vi "set FPS.vi"(8 "error in (no error)":errorcluster, 11 "Thorcam in":refnum<class "Thorcam.lvclass">) -> (0 "error out":errorcluster, 3 "Thorcam out":refnum<class "Thorcam.lvclass">)   [LabVIEW 2012, in "Thorcam.lvclass"]
uses:
  Thorcam.lvclass
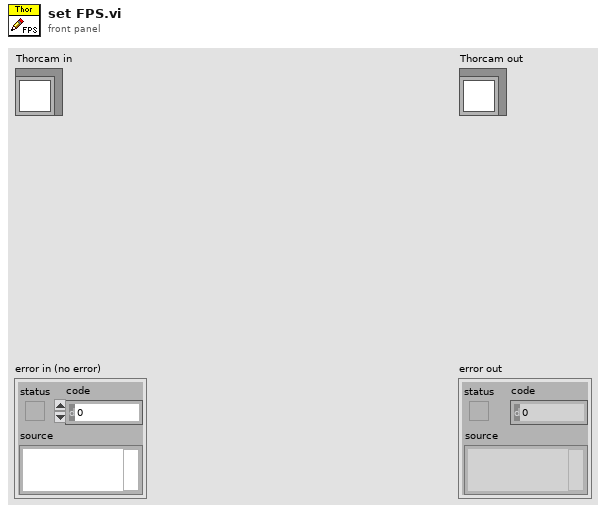
[diagram p1: front panel]
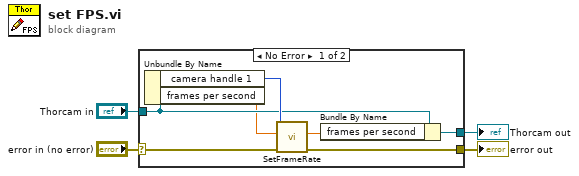
[diagram p0: block diagram]
diagram:
  n1 = case shown="No Error" "error in (no error)" {
    selector: "error in (no error)" -> [w10 w13]
    tunnel: [w9 w13] -> w3
    tunnel: [w7 w12] -> w1
    tunnel: "Thorcam in" -> [w8 w12]
    frame No Error {
      n2 = Unbundle By Name(w8) -> ("camera handle 1"=w11:u32, "frames per second"=w6:dbl)
      n3 = call <instrlib>:"SetFrameRate.vi"("error in"=w10, "FPS"=w6, "Camera Handle In"=w11) -> ("error out"=w9:errorcluster, "new FPS"=w5:dbl)  [unwired: 6 in, 1 out]
      n4 = Bundle By Name(cluster=w8, "frames per second"=w5) -> (w7:refnum<class "Thorcam.lvclass">)
    }
    frame Error {
    }
  }
  "error out" <- w3
  "Thorcam out" <- w1
